vi "WIRE_CLEAN_2 (SubVI).vi"(4 "Measured Output Value":dbl, 6 "Source":enum16{"Voltage", "Current"}(ring), 7 "string (\"\")":string, 9 "Numeric":dbl, 10 "string (\"\") 2":string, 11 "Measure (OUTPUT)":enum16{"Voltage", "Current"}(ring)) -> (1 "Array":dbl[](array[numeric]), 2 "String":string, 3 "output string 2":string, 5 "output string":string)   [LabVIEW 2020]
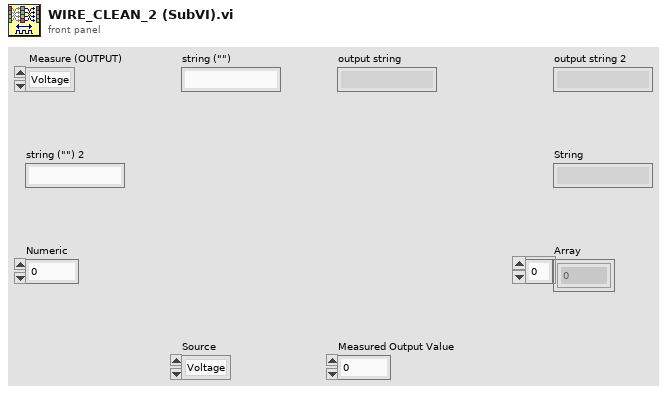
[diagram p1: front panel]
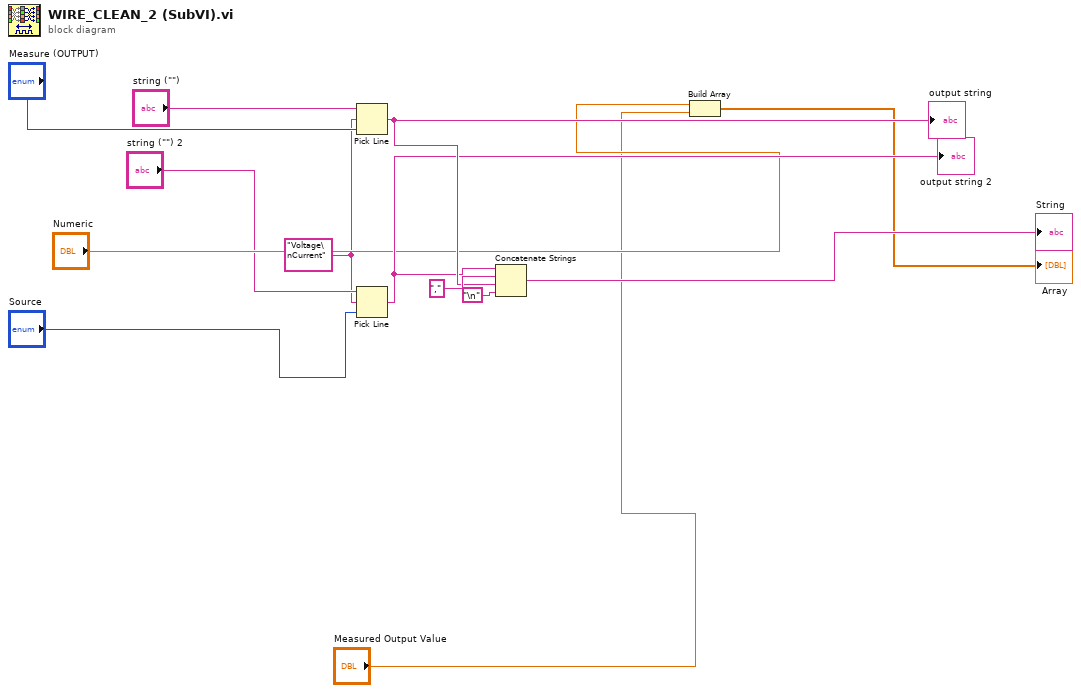
[diagram p0: block diagram]
diagram:
  w1 = "Voltage\nCurrent" ("multi-line string")
  n1 = Pick Line(string ("")="string (\"\")", multi-line string=w1, line index="Measure (OUTPUT)") -> (output string=w10:string)
  "output string" <- w10
  n2 = Pick Line(string ("")="string (\"\") 2", multi-line string=w1, line index="Source") -> (output string=w9:string)
  "output string 2" <- w9
  n3 = Concatenate Strings(w9, "," ("string"), w10, "\n") -> (→"String":string)
  n4 = Build Array("Numeric", "Measured Output Value") -> (→"Array":dbl[])
